vi "Pie Constructor.vi"(4 "Plot ID":i32, 8 "error in (no error)":errorcluster, 9 "offset vector":sgl[](array[numeric]), 10 "x vector":sgl[](array[numeric]), 11 "3D Quiver Datatype.lvclass in":refnum<class "3D Pie Datatype.lvclass">) -> (0 "error out":errorcluster, 3 "3D Quiver Datatype.lvclass out":refnum<class "3D Pie Datatype.lvclass">)   [LabVIEW 2017, in "3D Pie Datatype.lvclass"]
uses:
  <vilib>/Math Plots/3D Math Plots/3D Pie/3D Pie Datatype/3D Pie Datatype.lvclass
  <vilib>/Math Plots/3D Math Plots/3D Pie/3D Pie Datatype/3D Pie Datatype.lvclass/3D Pie Datatype.ctl
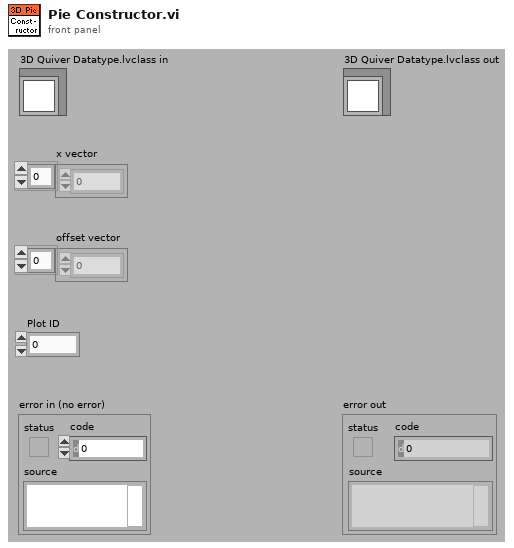
[diagram p1: front panel]
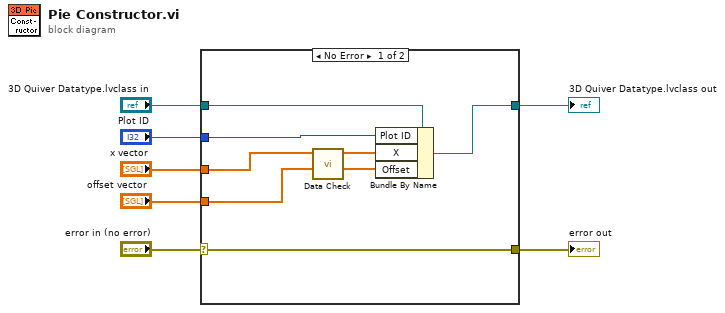
[diagram p0: block diagram]
diagram:
  n1 = case shown="No Error" "error in (no error)" {
    selector: "error in (no error)" -> [w13 w17]
    tunnel: "Plot ID" -> [w8 _]
    tunnel: [w13 w17] -> w6
    tunnel: "x vector" -> [w12 _]
    tunnel: "offset vector" -> [w9 _]
    tunnel: "3D Quiver Datatype.lvclass in" -> [w15 w16]
    tunnel: [w14 w16] -> w1
    frame No Error {
      n2 = call <vilib>:"Data Check.vi"("Offset In"=w9, "X In"=w12) -> ("Offset Out"=w10:sgl[], "X Out"=w11:sgl[])  [unwired: 1 in, 7 out]
      n3 = Bundle By Name(cluster=w15, "Plot ID"=w8, "X"=w11, "Offset"=w10) -> (w14:refnum<class "3D Pie Datatype.lvclass">)
    }
    frame Error {
    }
  }
  "error out" <- w6
  "3D Quiver Datatype.lvclass out" <- w1
